vi "mainControls.vi"(8 "error in (no error)":errorcluster, 11 "View in":refnum<class "View.lvclass">) -> (0 "error out":errorcluster, 3 "View out":refnum<class "View.lvclass">)   [LabVIEW 2015, in "View.lvclass"]
uses:
  View.lvclass
panel:
  in  "standby":bool
  in  "exitControl":bool
  in  "disable":bool
  in  "enable":bool
  in  "start":bool
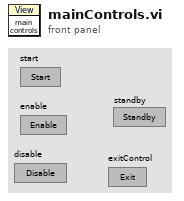
[diagram p1: front panel]
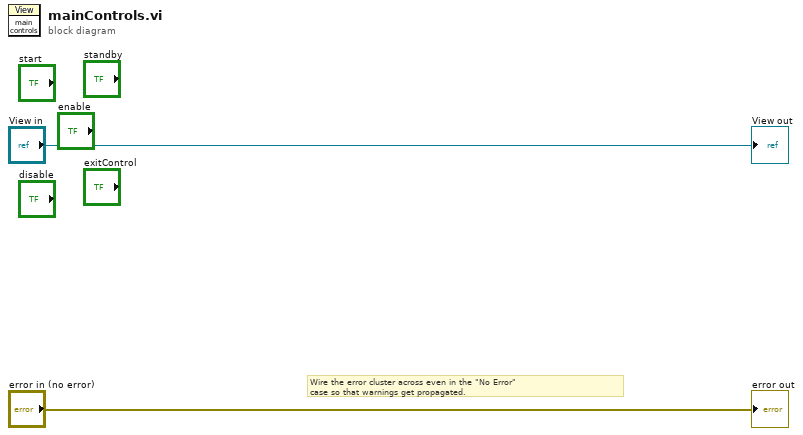
[diagram p0: block diagram]
diagram:
  # "Wire the error cluster across even in the \"No Error\"\ncase so that warnings get propagated."
  "error out" <- "error in (no error)"
  "View out" <- "View in"
